vi "Model Initial Values - Select Model Dialog.vi"(4 "Get Children?":bool, 6 "Multi-Selection?":bool, 7 "References?":bool, 8 "error in (no error)":errorcluster, 9 "Allow Section Selection (F)":bool, 10 "Initial Selection":T1[](array[typedef]) format="%.0x", 11 "Root Item Ref":T1 format="%.0x") -> (0 "error out":errorcluster, 1 "Canceled":bool, 3 "Selected Channel Refs":T1[](array[typedef]) format="%.0x")   [LabVIEW 2011, in "Model Initial Values Custom Device.lvlib"]
doc: "Standard Channel Select Dialog that allows the user to select which TimeStamp channel to use for the header information."
uses:
  Model Initial Values Custom Device.lvlib
  <vilib>/NI Veristand/Custom Device API/Custom Device Item Ref.ctl
  Model Initial Values - Global.vi
  <vilib>/NI Veristand/Custom Device API/Custom Device API.lvlib
  <vilib>/NI Veristand/Custom Device Tools/Custom Device Utility Library/Custom Device Utility Library.lvlib
panel:
  in  "Channels":string[](tree)
  in  "Cancel":bool
  in  "OK":bool
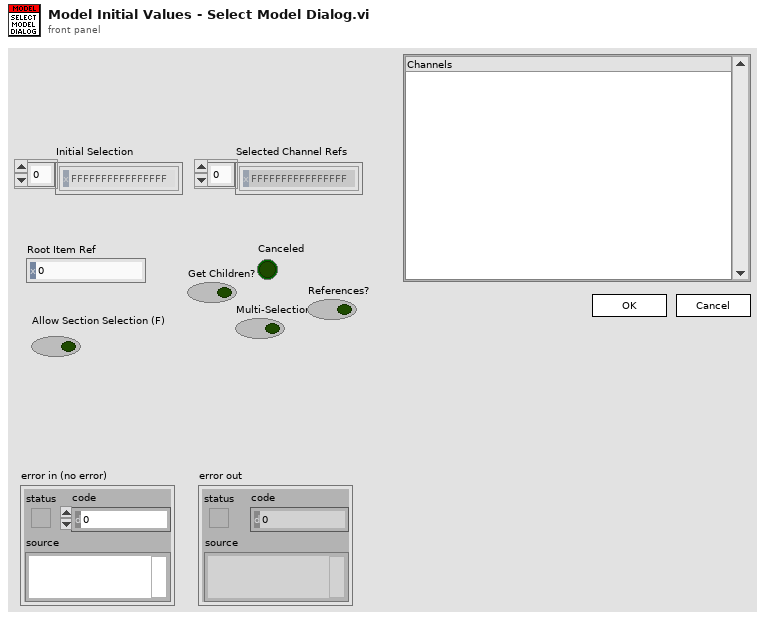
[diagram p1: front panel]
types:
  T1 = typedef "Custom Device API.lvlib/Custom Device Item Ref.ctl" = u64
  T2 = enum16{"Open or Add", "Close Ref", "Reset Local Store"}
  T3 = typedef "Custom Device API.lvlib/Custom Device Item Info.ctl" = cluster{"Name":string, "Is Channel":bool, "GUID":string}
  T4 = cluster{"Name":string, "Is Channel":bool, "GUID":string}
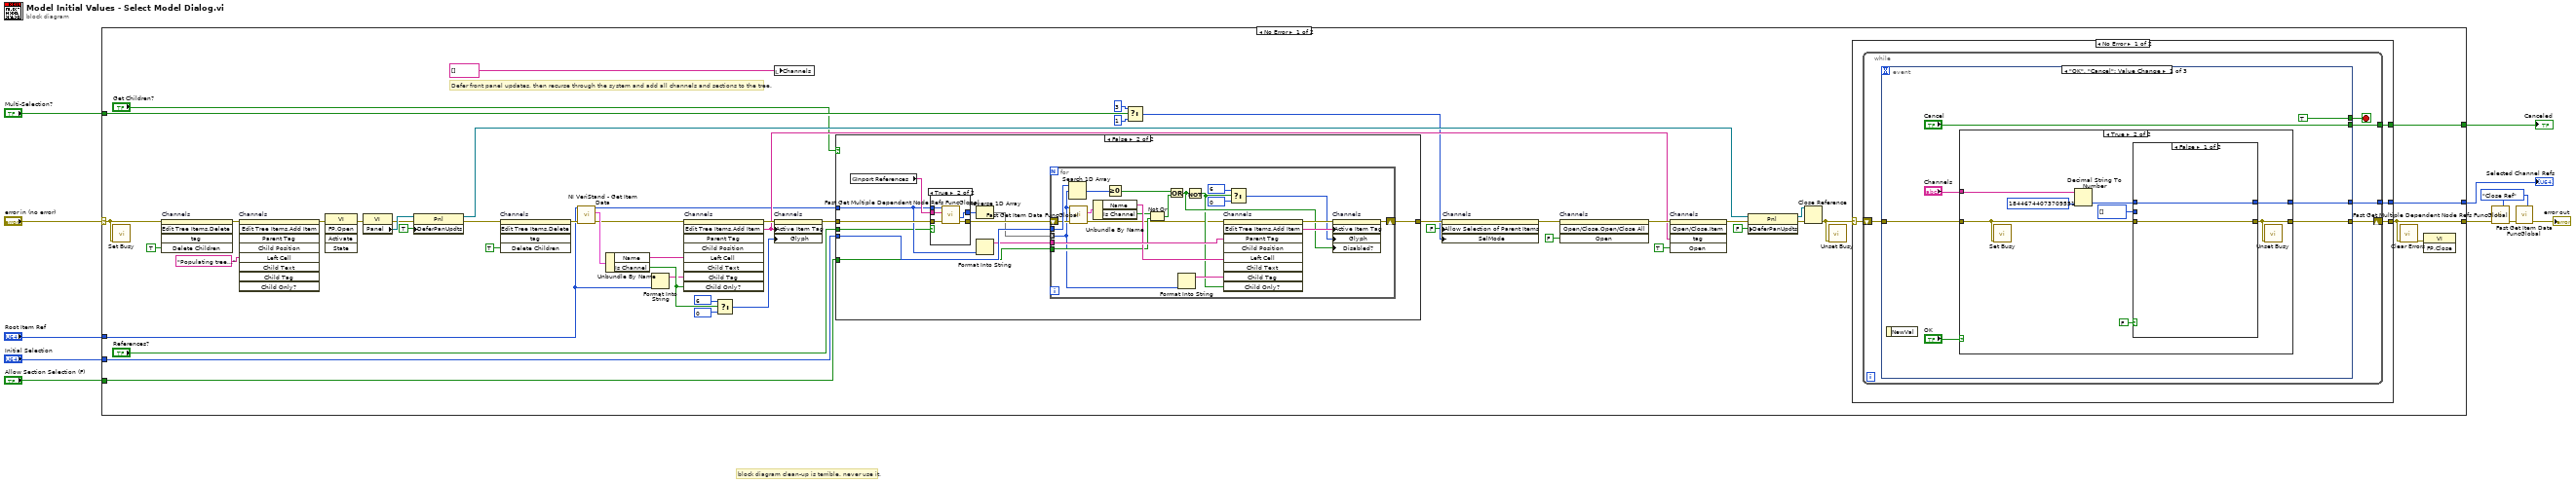
[diagram p0: block diagram]
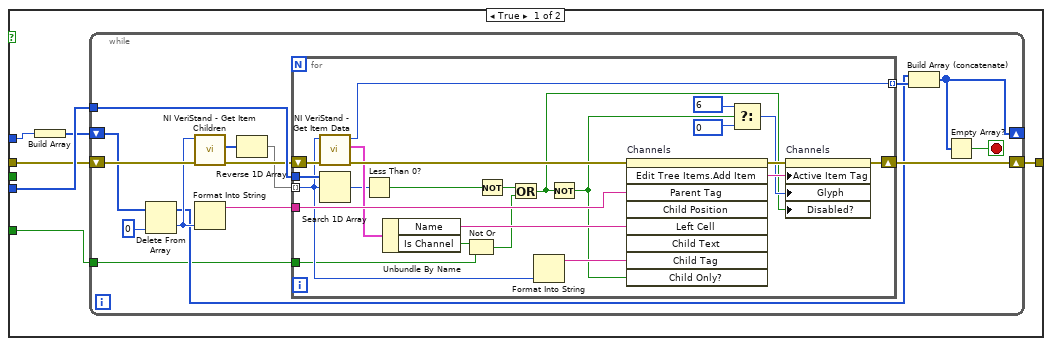
[diagram p2: hidden frame]
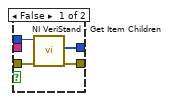
[diagram p3: hidden frame]
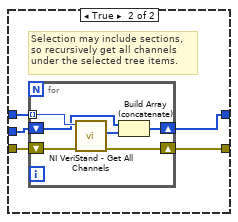
[diagram p5: hidden frame]
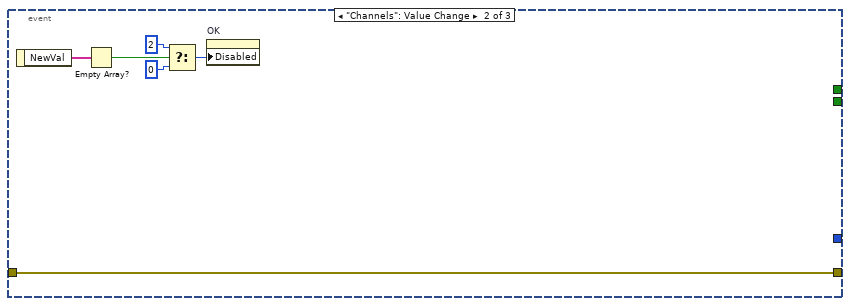
[diagram p6: hidden frame]
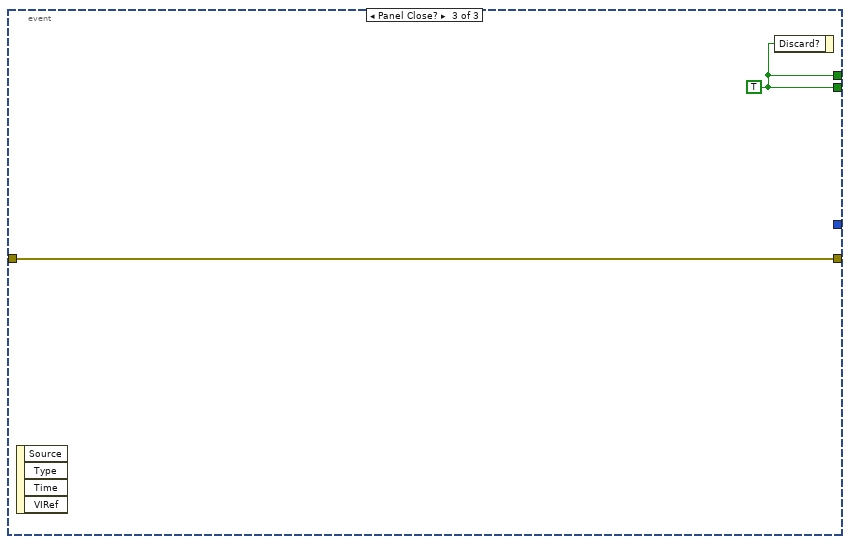
[diagram p7: hidden frame]
diagram:
  w2 = T2."Close Ref" ("Action")
  # "block diagram clean-up is terrible. never use it."
  n1 = case shown="No Error" "error in (no error)" {
    selector: "error in (no error)" -> [w23 w194]
    tunnel: "Initial Selection" -> [w25 _]
    tunnel: "Allow Section Selection (F)" -> [w13 _]
    tunnel: [w45 w194] -> w4
    tunnel: [w46 _] -> w8
    tunnel: [w43 _] -> w7
    tunnel: "Root Item Ref" -> [w24 _]
    tunnel: "Multi-Selection?" -> [w19 _]
    frame No Error {
      # "Defer front panel updates, then recurse through the system and add all channels and sections to the tree."
      n2 = call <vilib>:"Set Busy.vi"("error in (no error)"=w23) -> ()  [unwired: 3 in, 8 out]
      n3 = invoke on="Channels" class="Tree (strict)" method="Edit Tree Items.Delete"(error in=w23, "Delete Children"=TRUE ("Delete Children?")) -> (error out=w61:errorcluster)  [unwired: 3 in, 4 out]
      n4 = invoke on="Channels" class="Tree (strict)" method="Edit Tree Items.Add Item"(error in=w61, "Left Cell"="Populating tree..." ("Tag")) -> (error out=w58:errorcluster)  [unwired: 7 in, 8 out]
      n5 = invoke class="VI" method="FP.Open"(error in=w58) -> (error out=w56:errorcluster)  [unwired: 4 in, 4 out]
      n6 = property class="VI"(error in=w56) -> (error out=w54:errorcluster, "Panel"=w55:refnum<vi>)  [unwired: 1 in, 1 out]
      n7 = property class="Pnl"(reference=w55, error in=w54, "DeferPanUpdts"=TRUE ("Defer Panel Updates")) -> (reference out=w49:refnum<vi>, error out=w52:errorcluster)
      n8 = invoke on="Channels" class="Tree (strict)" method="Edit Tree Items.Delete"(error in=w52, "Delete Children"=TRUE ("Delete Children?")) -> (error out=w33:errorcluster)  [unwired: 3 in, 4 out]
      n9 = call <vilib>:"NI VeriStand - Get Item Data.vi"("error in (no error)"=w33, "Item Ref in"=w24) -> ("error out"=w34:errorcluster, "Item Info"=w36:T3, "Item Ref out"=w16:T1)  [unwired: 7 out]
      n10 = Unbundle By Name(w36) -> ("Name"=w37:string, "Is Channel"=w41:bool)
      n11 = Format Into String(w24) -> (resulting string=w35:string)  [unwired: 3 in, 1 out]
      n12 = invoke on="Channels" class="Tree (strict)" method="Edit Tree Items.Add Item"(error in=w34, "Left Cell"=w37, "Child Tag"=w35, "Child Only?"=w41) -> (error out=w38:errorcluster, "Edit Tree Items:Add Item"=w28:string)  [unwired: 5 in, 7 out]
      n13 = Select(t=6, s=w41, f=0) -> (s? t:f=w42:i32)
      n14 = local write "Channels"(string[] [] ("Channels")) -> ()
      n15 = property on="Channels" class="Tree (strict)"(error in=w38, "Active Item Tag"=w28, "Glyph"=w42) -> (error out=w17:errorcluster)  [unwired: 1 in, 1 out]
      n16 = case shown="False" "Get Children?" {
        tunnel: [w67 w116] -> w51
        tunnel: w16 -> [w64 w109]
        tunnel: w25 -> [w66 w115]
        tunnel: w17 -> [w65 w112]
        tunnel: "References?" -> [_ w108]
        tunnel: w13 -> [w62 w106]
        frame True {
          n17 = Build Array(w64) -> (w63:T1[])
          n18 = while {
            tunnel: w66 -> [w81]
            shift-right: [w69] -> _
            shift-left: w63 -> [w76]
            shift-right: [w82] -> w67
            shift-left: w65 -> [w79]
            tunnel: w62 -> [w68]
            stop <- w70 stop-if-true
            n19 = Delete From Array(array=w76, index=0) -> (deleted portion=w73:T1, array with subset deleted=w71:T1[])  [unwired: 1 in]
            n20 = call <vilib>:"NI VeriStand - Get Item Children.vi"("error in (no error)"=w79, "Item Ref in"=w73) -> ("error out"=w78:errorcluster, "Child Refs"=w80:T1[])  [unwired: 8 out]
            n21 = Format Into String(w73) -> (resulting string=w75:string)  [unwired: 3 in, 1 out]
            n22 = Reverse 1D Array(array=w80) -> (reversed array=w77:T1[])
            n23 = for {
              shift-right: [w97] -> w82
              shift-left: w78 -> [w104]
              tunnel: w77 -> [w92] mode=indexing
              tunnel: w75 -> [w105]
              tunnel: w81 -> [w93]
              tunnel: [w90] -> w74 mode=indexing
              tunnel: w68 -> [w85]
              n24 = call <vilib>:"NI VeriStand - Get Item Data.vi"("error in (no error)"=w104, "Item Ref in"=w92) -> ("error out"=w103:errorcluster, "Item Info"=w101:T3, "Item Ref out"=w90:T1)  [unwired: 7 out]
              n25 = Search 1D Array(1D array=w93, element=w92) -> (index of element=w91:i32)  [unwired: 1 in]
              n26 = Less Than 0?(x=w91) -> (x < 0?=w88:bool)
              n27 = Unbundle By Name(w101) -> ("Name"=w100:string, "Is Channel"=w87:bool)
              n28 = Not Or(1:w85, 2:w87) -> (0:w86:bool)
              n29 = Not(x=w88) -> (.not. x?=w89:bool)
              n30 = Or(x=w89, y=w86) -> (x .or. y?=w84:bool)
              n31 = Format Into String(w92) -> (resulting string=w102:string)  [unwired: 3 in, 1 out]
              n32 = Not(x=w84) -> (.not. x?=w83:bool)
              n33 = invoke on="Channels" class="Tree (strict)" method="Edit Tree Items.Add Item"(error in=w103, "Parent Tag"=w105, "Left Cell"=w100, "Child Tag"=w102, "Child Only?"=w83) -> (error out=w99:errorcluster, "Edit Tree Items:Add Item"=w98:string)  [unwired: 4 in, 7 out]
              n34 = Select(t=6, s=w83, f=0) -> (s? t:f=w94:i32)
              n35 = property on="Channels" class="Tree (strict)"(error in=w99, "Active Item Tag"=w98, "Glyph"=w94, "Disabled?"=w84) -> (error out=w97:errorcluster)  [unwired: 1 in, 1 out]
            }
            n36 = Build Array (concatenate)(w71, w74) -> (w69:T1[])
            n37 = Empty Array?(array=w69) -> (empty?=w70:bool)
          }
        }
        frame False {
          n38 = global read "Model Initial Values - Global.vi" "Inport References"() -> (w113:string)
          n39 = case shown="True" w108 {
            tunnel: w112 -> [w120 w125]
            tunnel: [w119 w124] -> w111
            tunnel: [w118 w123] -> w114
            tunnel: w109 -> [w117 w121]
            tunnel: w113 -> [_ w122]
            frame False {
              n40 = call <vilib>:"NI VeriStand - Get Item Children.vi"("error in (no error)"=w120, "Item Ref in"=w117) -> ("error out"=w119:errorcluster, "Child Refs"=w118:T1[])  [unwired: 8 out]
            }
            frame True {
              n41 = call "Fast Get Multiple Dependent Node Refs FuncGlobal.vi"("error in (no error)"=w125, "Base Property Name"=w122, "Item Ref in"=w121) -> ("error out"=w124:errorcluster, "Dependent Node Refs"=w123:T1[])  [unwired: 6 in, 1 out]
            }
          }
          n42 = Reverse 1D Array(array=w114) -> (reversed array=w110:T1[])
          n43 = Format Into String(w109) -> (resulting string=w107:string)  [unwired: 3 in, 1 out]
          n44 = for {
            shift-right: [w141] -> w116
            shift-left: w111 -> [w129]
            tunnel: w110 -> [w126] mode=indexing
            tunnel: w107 -> [w146]
            tunnel: w115 -> [w137]
            tunnel: w106 -> [w133]
            n45 = Search 1D Array(1D array=w137, element=w126) -> (index of element=w136:i32)  [unwired: 1 in]
            n46 = call "Fast Get Item Data FuncGlobal.vi"("error in (no error)"=w129, "Item Ref in"=w126) -> ("error out"=w128:errorcluster, "Item Info"=w127:T4)  [unwired: 6 in, 2 out]
            n47 = Unbundle By Name(w127) -> ("Name"=w144:string, "Is Channel"=w132:bool)
            n48 = Greater Or Equal To 0?(x=w136) -> (x >= 0?=w130:bool)
            n49 = Not Or(1:w133, 2:w132) -> (0:w135:bool)
            n50 = Or(x=w130, y=w135) -> (x .or. y?=w134:bool)
            n51 = Format Into String(w126) -> (resulting string=w145:string)  [unwired: 3 in, 1 out]
            n52 = Not(x=w134) -> (.not. x?=w131:bool)
            n53 = invoke on="Channels" class="Tree (strict)" method="Edit Tree Items.Add Item"(error in=w128, "Parent Tag"=w146, "Left Cell"=w144, "Child Tag"=w145, "Child Only?"=w131) -> (error out=w143:errorcluster, "Edit Tree Items:Add Item"=w142:string)  [unwired: 4 in, 7 out]
            n54 = Select(t=6, s=w131, f=0) -> (s? t:f=w138:i32)
            n55 = property on="Channels" class="Tree (strict)"(error in=w143, "Active Item Tag"=w142, "Glyph"=w138, "Disabled?"=w134) -> (error out=w141:errorcluster)  [unwired: 1 in, 1 out]
          }
        }
      }
      n56 = Select(t=3 ("Selection Mode"), s=w19, f=1 ("Selection Mode")) -> (s? t:f=w20:i32)
      n57 = property on="Channels" class="Tree (strict)"(error in=w51, "Allow Selection of Parent Items"=FALSE, "SelMode"=w20) -> (error out=w32:errorcluster)  [unwired: 1 in, 1 out]
      n58 = invoke on="Channels" class="Tree (strict)" method="Open/Close.Open/Close All"(error in=w32, "Open"=FALSE ("Open?")) -> (error out=w30:errorcluster)  [unwired: 2 in, 3 out]
      n59 = invoke on="Channels" class="Tree (strict)" method="Open/Close.Item"(error in=w30, "tag"=w28, "Open"=TRUE ("Open?")) -> (error out=w26:errorcluster)  [unwired: 2 in, 4 out]
      n60 = property class="Pnl"(reference=w49, error in=w26, "DeferPanUpdts"=FALSE ("Defer Panel Updates")) -> (reference out=w47:refnum<vi>, error out=w48:errorcluster)
      n61 = Close Reference(reference=w47, error in (no error)=w48) -> (error out=w27:errorcluster)
      n62 = call <vilib>:"Unset Busy.vi"("error in (no error)"=w27) -> ()  [unwired: 1 in, 10 out]
      n63 = case shown="No Error" w27 {
        selector: w27 -> [w150 w193]
        tunnel: [w149 w193] -> w45
        tunnel: [w148 _] -> w46
        tunnel: [w147 _] -> w43
        frame No Error {
          n64 = while {
            shift-right: [w154] -> w149
            shift-left: w150 -> [w155]
            tunnel: [w153] -> w148
            tunnel: [w151] -> w147
            stop <- w152 stop-if-true
            n65 = event shown="[0] \"OK\", \"Cancel\": Value Change" {
              selector: _ -> [_ _ _]
              dyn-events: _ -> [_ _ _]
              timeout: _ -> [_ _ _]
              tunnel: w155 -> [w159 w190 w192]
              tunnel: [w157 w190 w192] -> w154
              tunnel: ["Cancel" _ w191] -> w153
              tunnel: [TRUE ("Discard?") _ w191] -> w152
              tunnel: [w158 _ _] -> w151
              event "OK", "Cancel": Value Change {
                n66 = event-data() -> ()  [unwired: 2 out]
                n67 = case shown="True" "OK" {
                  tunnel: "Channels" -> [_ w171]
                  tunnel: w159 -> [w163 w165]
                  tunnel: [_ w169] -> w158
                  tunnel: [w163 w166] -> w157
                  frame False {
                  }
                  frame True {
                    n68 = call <vilib>:"Set Busy.vi"("error in (no error)"=w165) -> ()  [unwired: 3 in, 8 out]
                    n69 = Decimal String To Number(string=w171, default (0L)=T1 18446744073709551615 ("Device Item Ref")) -> (number=w168:u64[])  [unwired: 2 out]
                    n70 = case shown="False" FALSE {
                      tunnel: w165 -> [w172 w178]
                      tunnel: [w173 w176] -> w169
                      tunnel: w168 -> [w173 w175]
                      tunnel: [w172 w174] -> w166
                      tunnel: T1[] [] ("Channel Refs") -> [_ w177]
                      frame False {
                      }
                      frame True {
                        # "Selection may include sections, so recursively get all channels under the selected tree items."
                        n71 = for {
                          shift-right: [w180] -> w176
                          shift-left: w177 -> [w181]
                          shift-right: [w183] -> w174
                          shift-left: w178 -> [w184]
                          tunnel: w175 -> [w182] mode=indexing
                          n72 = call <vilib>:"NI VeriStand - Get All Channels.vi"("error in"=w184, "Section Ref in"=w182) -> ("error out"=w183:errorcluster, "Channel Refs"=w179:T1[])  [unwired: 8 out]
                          n73 = Build Array (concatenate)(w181, w179) -> (w180:T1[])
                        }
                      }
                    }
                    n74 = call <vilib>:"Unset Busy.vi"("error in (no error)"=w166) -> ()  [unwired: 1 in, 10 out]
                  }
                }
              }
              event "Channels": Value Change {
                n75 = event-data() -> ("NewVal"=w189:string[])  [unwired: 1 out]
                n76 = Empty Array?(array=w189) -> (empty?=w188:bool)
                n77 = Select(t=u8 2, s=w188, f=u8 0) -> (s? t:f=w185:u8)
                n78 = property on="OK" class="Bool"("Disabled"=w185) -> ()  [unwired: 2 in, 2 out]
              }
              event Panel Close? {
                w191 = TRUE ("Discard?")
                n79 = event-data() -> ()  [unwired: 5 out]
                n80 = event-data("Discard?"=w191) -> ()  [unwired: 1 in, 1 out]
              }
            }
          }
        }
        frame Error {
        }
      }
      n81 = call <vilib>:"Clear Errors.vi"("error in (no error)"=w45) -> ("error out"=w44:errorcluster)  [unwired: 6 out]
      n82 = invoke class="VI" method="FP.Close"(error in=w44) -> ()  [unwired: 2 in, 3 out]
    }
    frame Error {
    }
  }
  "Canceled" <- w8
  "Selected Channel Refs" <- w7
  n83 = call "Fast Get Multiple Dependent Node Refs FuncGlobal.vi"("Action"=w2, "error in (no error)"=w4) -> ("error out"=w3:errorcluster)  [unwired: 7 in, 2 out]
  n84 = call "Fast Get Item Data FuncGlobal.vi"("Action"=w2, "error in (no error)"=w3) -> ("error out"=→"error out":errorcluster)  [unwired: 6 in, 3 out]
